vi "Read Transfer Channels.vi"(8 "error in (no error)":errorcluster, 11 "E2E Tag Exchange configuration in":refnum<class "E2E Tag Exchange configuration.lvclass">) -> (0 "error out":errorcluster, 2 "Transfer Channels":refnum<class "TBM channel.lvclass">[](array[class]), 3 "E2E Tag Exchange configuration out":refnum<class "E2E Tag Exchange configuration.lvclass">)   [LabVIEW 2015]
uses:
  E2E Tag Exchange configuration.lvclass
  <vilib>/NI/Tag Bus Module Framework/channel/TBM channel.lvclass
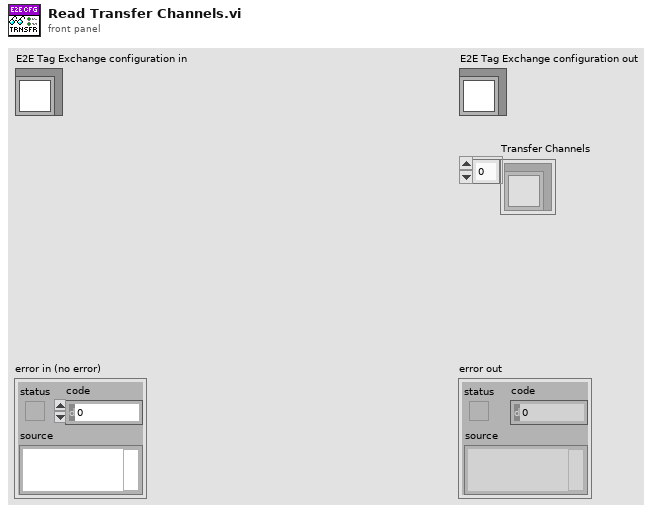
[diagram p1: front panel]
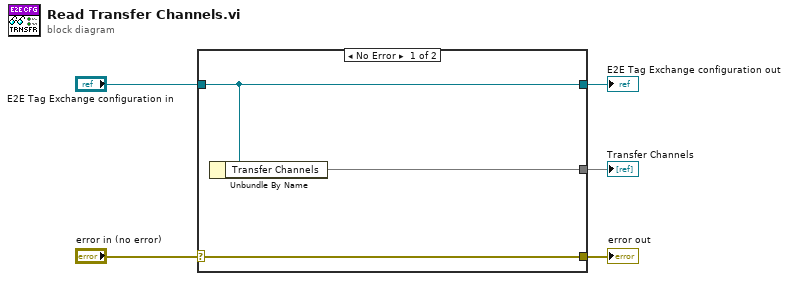
[diagram p0: block diagram]
diagram:
  n1 = case shown="No Error" "error in (no error)" {
    selector: "error in (no error)" -> [w8 w9]
    tunnel: [w8 w9] -> w4
    tunnel: [w7 w10] -> w2
    tunnel: "E2E Tag Exchange configuration in" -> [w7 w10]
    tunnel: [w6 _] -> w1
    frame No Error {
      n2 = Unbundle By Name(w7) -> ("Transfer Channels"=w6)
    }
    frame Error {
    }
  }
  "error out" <- w4
  "E2E Tag Exchange configuration out" <- w2
  "Transfer Channels" <- w1
